vi "Get_Class_Name.vi"(0 "File_Names":string[](array[string]), 11 "Error_In":errorcluster) -> (4 "Class_Names":string[](array[string]), 15 "Error_Out":errorcluster)   [LabVIEW 2023]
doc: "Used to get the class names"
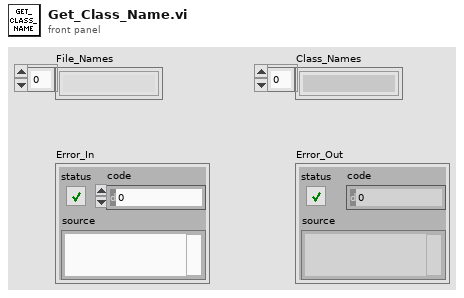
[diagram p1: front panel]
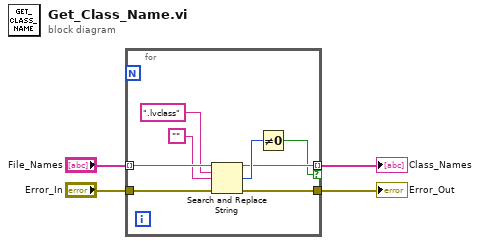
[diagram p0: block diagram]
diagram:
  n1 = for {
    tunnel: "Error_In" -> [w12]
    tunnel: [w11] -> w2
    tunnel: "File_Names" -> [w10] mode=indexing
    tunnel: [w6] -> w4 mode=indexing if=w5
    n2 = Search and Replace String(input string=w10, search string=".lvclass" ("input string"), replace string="", error in=w12) -> (result string=w6:string, number of replacements=w7:i32, error out=w11:errorcluster)  [unwired: 4 in, 1 out]
    n3 = Not Equal To 0?(x=w7) -> (x != 0?=w5:bool)
  }
  "Class_Names" <- w4
  "Error_Out" <- w2
